vi "polynomial fit.vi"() -> ()   [LabVIEW 2019]
uses:
  <vilib>/Analysis/NI_AALPro.lvlib
panel:
  out "XY Graph":cluster{i32[], dbl[]}[](graph)
  in  "days":i32[](array[numeric])
  in  "cumulative deaths":i32[](array[numeric])
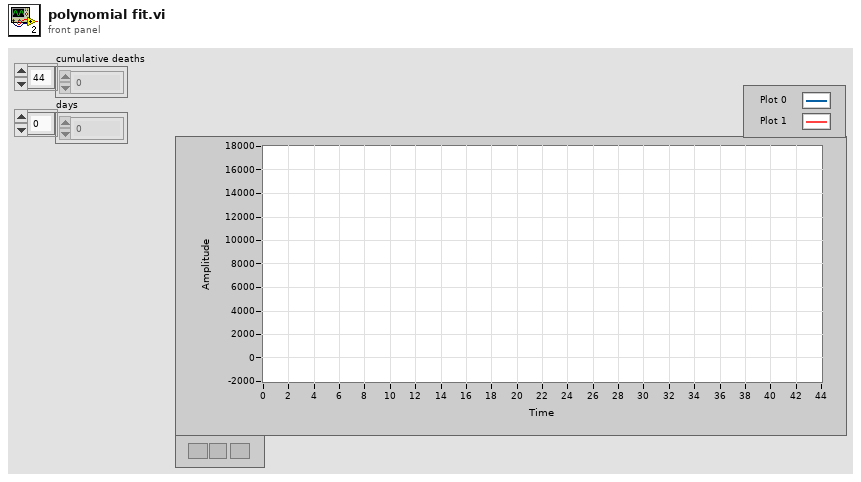
[diagram p1: front panel]
types:
  T1 = cluster{"days":i32[], "cumulative deaths":dbl[]}[]
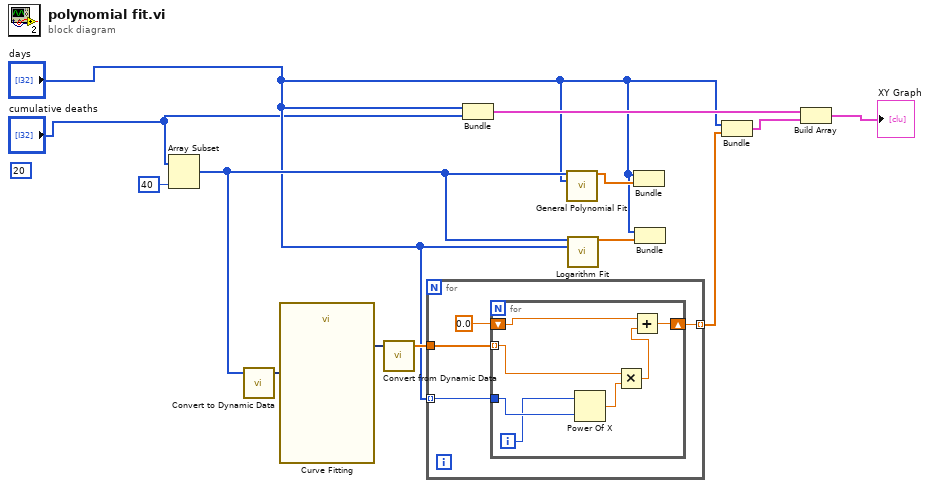
[diagram p0: block diagram]
diagram:
  (unwired) 20 ("index")
  n1 = Array Subset(array="cumulative deaths", length=40 ("index")) -> (w9:i32[])  [unwired: 1 in]
  n2 = call "Convert to Dynamic Data"("Array"=w9) -> ("Dynamic Data Type"=w8:dynamicdata)  [unwired: 3 in]
  n3 = call "Curve Fitting"("Signals"=w8) -> ("polynomial coefficients"=w7:dynamicdata)  [unwired: 6 in, 4 out]
  n4 = call "Convert from Dynamic Data"("Dynamic Data Type"=w7) -> ("Array"=w6:dbl[])  [unwired: 3 in]
  n5 = for {
    tunnel: w6 -> [w17]
    tunnel: "days" -> [w16] mode=indexing
    tunnel: [w15] -> w4 mode=indexing
    n6 = for {
      tunnel: w17 -> [w23] mode=indexing
      tunnel: w16 -> [w19]
      shift-right: [w22] -> w15
      shift-left: 0.0 -> [w20]
      i -> [w18]
      n7 = Power Of X(1:w19, 2:w18) -> (0:w24:dbl)
      n8 = Multiply(x=w23, y=w24) -> (x*y=w21:dbl)
      n9 = Add(x=w20, y=w21) -> (x+y=w22:dbl)
    }
  }
  n10 = Bundle("days"="days", "cumulative deaths"="cumulative deaths") -> (w13:cluster{"days":i32[], "cumulative deaths":i32[]})  [unwired: 1 in]
  n11 = call <vilib>:"General Polynomial Fit.vi"("Y"=w9, "X"="days") -> ("Best Polynomial Fit"=w11:dbl[])  [unwired: 10 in, 3 out]
  n12 = call <vilib>:"Logarithm Fit.vi"("Y"=w9, "X"="days") -> ("Best Logarithm Fit"=w10:dbl[])  [unwired: 9 in, 4 out]
  n13 = Bundle("days"="days", "Best Polynomial Fit"=w11) -> ()  [unwired: 1 in, 1 out]
  n14 = Bundle("days"="days", "Best Logarithm Fit"=w10) -> ()  [unwired: 1 in, 1 out]
  n15 = Bundle("days"="days", w4) -> (w5:cluster{"days":i32[], dbl[]})  [unwired: 1 in]
  n16 = Build Array(w13, w5) -> (→"XY Graph":T1)
